vi "Get Robot Pose.vi"(11 "robots":refnum<class "Robot.lvclass">) -> (3 "Pose":sgl[](array[numeric]))   [LabVIEW 2018]
uses:
  Robot_class/Robot.lvclass
  C:/Users/anton/Desktop/roboime/oop-vision/SSL_AI/Object_class/Object.lvclass
  Object_class/Object.lvclass/Object.ctl
  Robot_class/Robot.lvclass/Robot.ctl
  Object_class/Read x.vi
  Object_class/Read y.vi
  Robot_class/Read orientation.vi
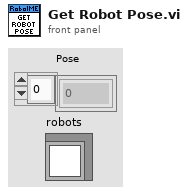
[diagram p1: front panel]
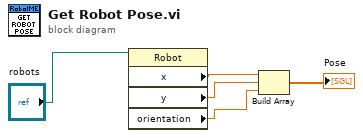
[diagram p0: block diagram]
diagram:
  n1 = property class="Robot"(reference="robots") -> ("x"=w3:dbl, "y"=w2:dbl, "orientation"=w1:dbl)  [unwired: 1 in, 2 out]
  n2 = Build Array(w3, w2, w1) -> (→"Pose":dbl[])
